vi "DB SPROC Param.vi"(8 "error in (no error)":errorcluster, 9 "Parameters":T1[](array[typedef])=[{"parameter name"="param1", "type"=enum."Long (I32)", "direction"=enum."Input", "value"=variant(i32 3)}], 10 "Stored Procedure":string="MultiplyAges", 11 "Connection Information":path=path "SQL.dsn") -> (0 "error out":errorcluster, 3 "Recordset Data":string[][](table))   [LabVIEW 2011]
doc: "Executes a stored procedure on the database passed in.\n\n<b>Connection Information</b> - Path to the file DSN for connection to the ODBC database.\n\n<b>Stored Procedure</b> - Name of the stored procedure to execute.\n\n<b>Parameters (optional)</b> - Parameters to pass to the stored procedure.\n\n\nVersion 1.0 - 10/20/2009\n\nPhaeron, Inc.\nwww.phaeron.com\ninfo@phaeron.com"
uses:
  <vilib>/addons/database/NI_Database_API.lvlib
  <vilib>/addons/database/_DB Variant To Data/Database Variant To Data.xnode
  <vilib>/addons/database/Command.llb/Cmd Execute.vi
  <vilib>/addons/database/Recordset.llb/Rec Fetch Recordset Data (CR).vi
  <vilib>/addons/database/Recordset.llb/Rec Destroy - Command.vi
  <vilib>/addons/database/Command.llb/Cmd Delete.vi
  <vilib>/addons/database/Connection.llb/DB Tools Open Connec (Path).vi
  <vilib>/addons/database/Auxilliary.llb/DB Tools DataTypes.ctl
  <vilib>/addons/database/Auxilliary.llb/DB Tools Parameter Dir.ctl
  <vilib>/addons/database/Auxilliary.llb/DB Tools Parameter Info.ctl
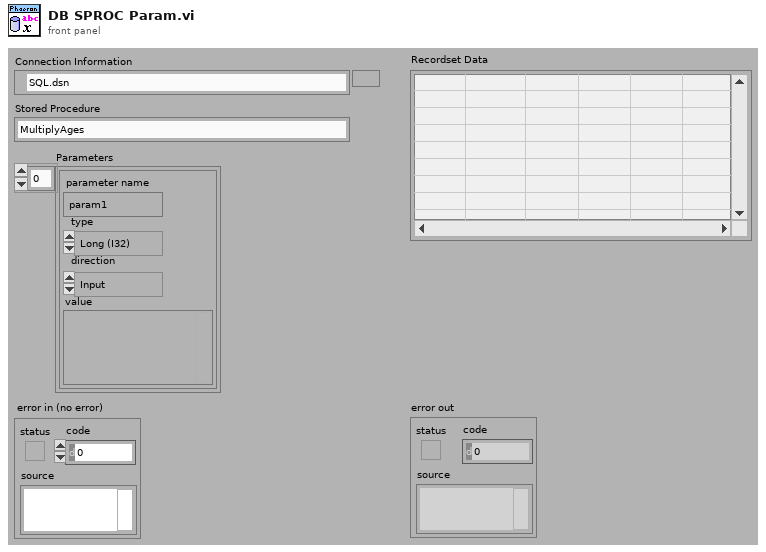
[diagram p1: front panel]
types:
  T1 = typedef "NI_Database_API.lvlib/DB Tools Parameter Info.ctl" = cluster{"parameter name":string, "type":T2, "direction":T3, "value":variant}
  T2 = typedef "NI_Database_API.lvlib/DB Tools DataTypes.ctl" = enum16{"String", "Long (I32)", "Single (SGL)", "Double (DBL)", "Date/Time", "Binary"}
  T3 = typedef "NI_Database_API.lvlib/DB Tools Parameter Dir.ctl" = enum32{"Input", "Output", "Input/Output", "Return Value"}
  T4 = typedef "NI_Database_API.lvlib/Conn ObjectReference.ctl" = refnum<k1>
  T5 = typedef "NI_Database_API.lvlib/Cmd ObjectReference.ctl" = refnum<k1>
  T6 = typedef "NI_Database_API.lvlib/Cmd-Rec Object Reference.ctl" = refnum<k1>
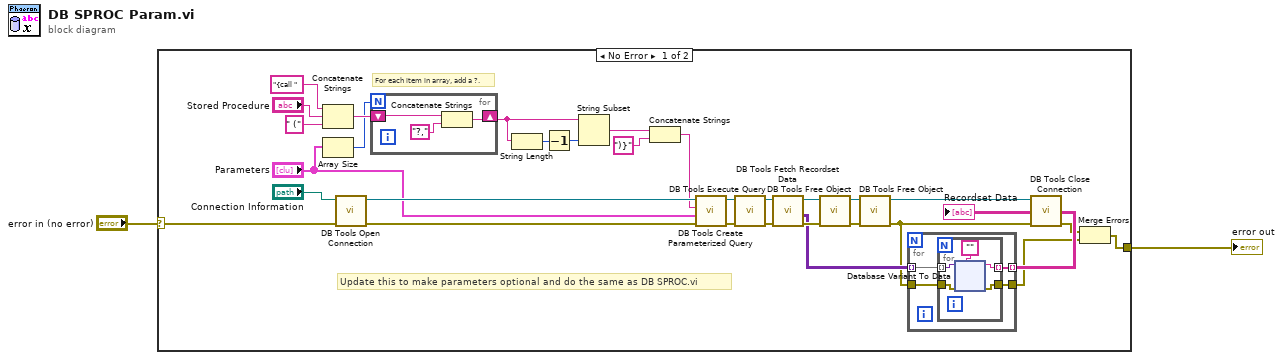
[diagram p0: block diagram]
diagram:
  n1 = case shown="No Error" "error in (no error)" {
    selector: "error in (no error)" -> [w3 w78]
    tunnel: [w16 w78] -> w2
    frame No Error {
      # "Update this to make parameters optional and do the same as DB SPROC.vi"
      # "For each item in array, add a ?."
      n2 = Concatenate Strings("{call " ("SQL query 2"), "Stored Procedure", " (" ("SQL query 2")) -> (w12:string)
      n3 = Array Size(array="Parameters") -> (size(s)=w7:i32)
      n4 = call-poly <vilib>:"DB Tools Open Connection.vi"("error in (no error)"=w3, "connection information"="Connection Information") -> ("error out"=w26:errorcluster, "connection reference"=w25:T4)  [unwired: 6 in]
      n5 = for {
        N: w7 -> [_]
        shift-right: [w34] -> w11
        shift-left: w12 -> [w36]
        n6 = Concatenate Strings(w36, "?,") -> (w34:string)
      }
      n7 = String Length(string=w11) -> (length=w10:i32)
      n8 = Decrement(x=w10) -> (x-1=w9:i32)
      n9 = String Subset(string=w11, length (rest)=w9) -> (substring=w6:string)  [unwired: 1 in]
      n10 = Concatenate Strings(w6, ")}" ("SQL query 2")) -> (w5:string)
      n11 = call <vilib>:"DB Tools Create Parameterized Query.vi"("error in (no error)"=w26, "parameters"="Parameters", "SQL query"=w5, "connection reference"=w25) -> ("error out"=w24:errorcluster, "command reference"=w23:T5)  [unwired: 3 in, 1 out]
      n12 = call-poly <vilib>:"DB Tools Execute Query.vi"("error in (no error)"=w24, "command reference"=w23) -> ("error out"=w31:errorcluster, "command-recordset reference"=w33:T6)  [unwired: 6 in]
      n13 = call-poly <vilib>:"DB Tools Fetch Recordset Data.vi"("error in (no error)"=w31, "command-recordset reference"=w33) -> ("error out"=w29:errorcluster, "recordset data"=w27:variant[][], "command-recordset reference out"=w30:T6)  [unwired: 3 in]
      n14 = call-poly <vilib>:"DB Tools Free Object.vi"("error in (no error)"=w29, "command-recordset reference"=w30) -> ("error out"=w20:errorcluster, "command reference"=w22:T5)  [unwired: 8 in]
      n15 = call-poly <vilib>:"DB Tools Free Object.vi"("error in (no error)"=w20, "command reference"=w22) -> ("error out"=w19:errorcluster, "connection reference"=w21:T4)  [unwired: 8 in]
      n16 = for {
        tunnel: [w40] -> w28 mode=indexing
        tunnel: w27 -> [w39] mode=indexing
        tunnel: w19 -> [w38]
        tunnel: [w37] -> w17
        n17 = for {
          tunnel: [w44] -> w40 mode=indexing
          tunnel: w39 -> [w43] mode=indexing
          tunnel: w38 -> [w42]
          tunnel: [w41] -> w37
          n18 = xnode "Database Variant To Data"("database variant"=w43, "error in"=w42, "type"="") -> ("data"=w44:string, "error out"=w41:errorcluster)
        }
      }
      "Recordset Data" <- w28
      n19 = call <vilib>:"DB Tools Close Connection.vi"("error in (no error)"=w19, "connection reference"=w21) -> ("error out"=w18:errorcluster)  [unwired: 5 in]
      n20 = Merge Errors(w18, w17) -> (w16:errorcluster)
    }
    frame Error {
    }
  }
  "error out" <- w2
